vi "Swerve Drive.vi"(5 "Rot. Point X":dbl, 6 "Auto Controls":bool, 7 "Rot. Point Y":dbl) -> ()   [LabVIEW 2020]
uses:
  Robot Global Data.vi
  <vilib>/addons/control/pid/pid.llb/PID (DBL).vi
  <vilib>/addons/control/pid/NI_PID_pid.lvlib
panel:
  out "Gyro Angle":dbl(knob)=-0.120849609375 scale=0.0..360.0
  out "Heading":dbl=-0.60150146484375
  in  "Maintain Z Angle PID gains":T1={"proportional gain (Kc)"=0.0045, "integral time (Ti, min)"=0.0, "derivative time (Td, min)"=0.0} {"derivative time (Td, min)" format="%.4f"; "integral time (Ti, min)" format="%.4f"; "proportional gain (Kc)" format="%.4f"}
  in  "FeedForward":dbl
  in  "fr offset":dbl(knob)=326.0 scale=-180.0..180.0
  in  "fl offset":dbl(knob)=182.3 scale=-180.0..180.0
  in  "br offset":dbl(knob)=52.0 scale=-180.0..180.0
  in  "bl offset":dbl(knob)=358.0 scale=-180.0..180.0
  in  "Robot Length":dbl=25.0
  in  "Robot Width":dbl=25.0
  # "Comp bot\nFL: -2\nFR: -2\nBL: -1\nBR: 0"
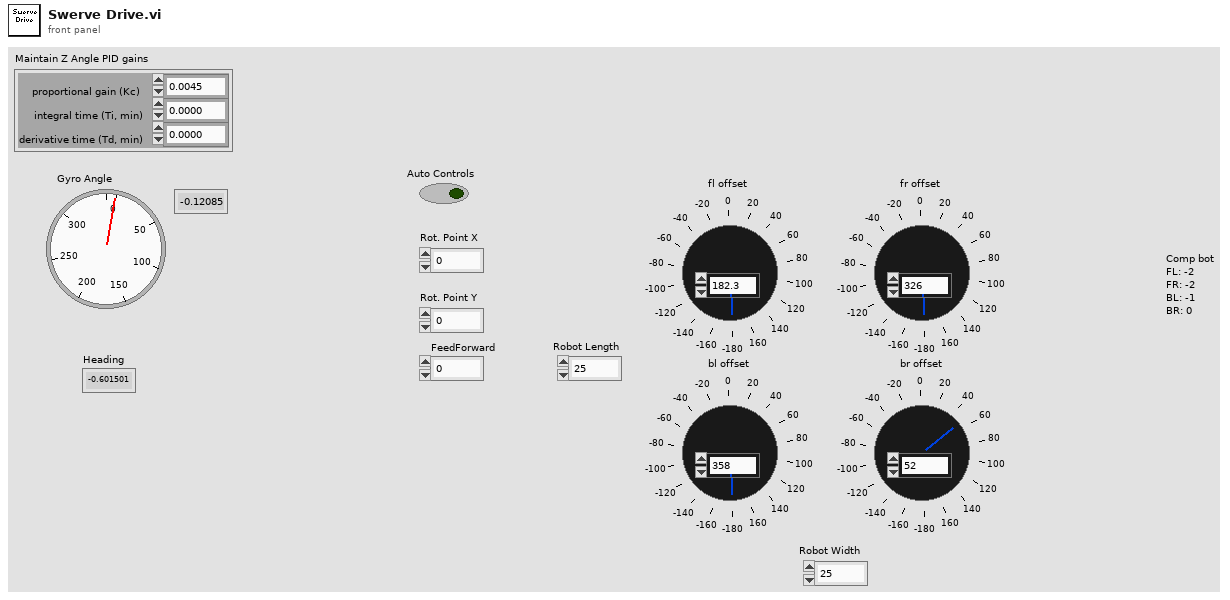
[diagram p1: front panel]
types:
  T1 = cluster{"proportional gain (Kc)":dbl, "integral time (Ti, min)":dbl, "derivative time (Td, min)":dbl}
  T2 = enum16{"Back Left", "Back Right", "Front Left", "Front Right"}
  T3 = typedef "WPI_MotorControlDeviceRef.ctl" = cluster{"DeviceStatus":errorcluster, "Type":T4, "PWM":cluster{"PWM Channel":T5, "DeadBand":T6}, "CAN":cluster{"Device Number":u8, "SetOutput VI Ref":variant, "GetOutput VI Ref":variant, "Enable VI Ref":variant, "Disable VI Ref":variant, "Data":variant}, "Invert":bool, "DIO PWM":cluster{"PWM \"Enable\" Channel":T5, "DIOChannel":T7, "PWM Rate":dbl}}
  T4 = typedef "WPI_MotorControlType.ctl" = enum16{"PWM", "CAN", "DIO PWM"}
  T5 = typedef "FPGA_DIOPWMChannel.ctl" = enum8{"PWM 0", "PWM 1", "PWM 2", "PWM 3", "PWM 4", "PWM 5", "PWM 6", "PWM 7", "PWM 8", "PWM 9", "PWM MXP 0", "PWM MXP 1", "PWM MXP 2", "PWM MXP 3", "PWM MXP 4", "PWM MXP 5", "PWM MXP 6", "PWM MXP 7", "PWM MXP 8", "PWM MXP 9", "Invalid"}
  T6 = typedef "WPI_PWMDeadband.ctl" = cluster{"Name":string, "maxPositivePwm":i32, "minPositivePwm":i32, "centerPwm":i32, "maxNegativePwm":i32, "minNegativePwm":i32, "angularRange":u16}
  T7 = typedef "FPGA_DIOChannel.ctl" = enum8{"DIO 0", "DIO 1", "DIO 2", "DIO 3", "DIO 4", "DIO 5", "DIO 6", "DIO 7", "DIO 8", "DIO 9", "DIO MXP 0", "DIO MXP 1", "DIO MXP 2", "DIO MXP 3", "DIO MXP 4", "DIO MXP 5", "DIO MXP 6", "DIO MXP 7", "DIO MXP 8", "DIO MXP 9", "DIO MXP 10", "DIO MXP 11", "DIO MXP 12", "DIO MXP 13", "DIO MXP 14", "DIO MXP 15", "SPI Port CS1", "SPI Port CS2", "SPI Port CS3", "SPI Port MISO", "SPI Port MOSI", "Invalid"}
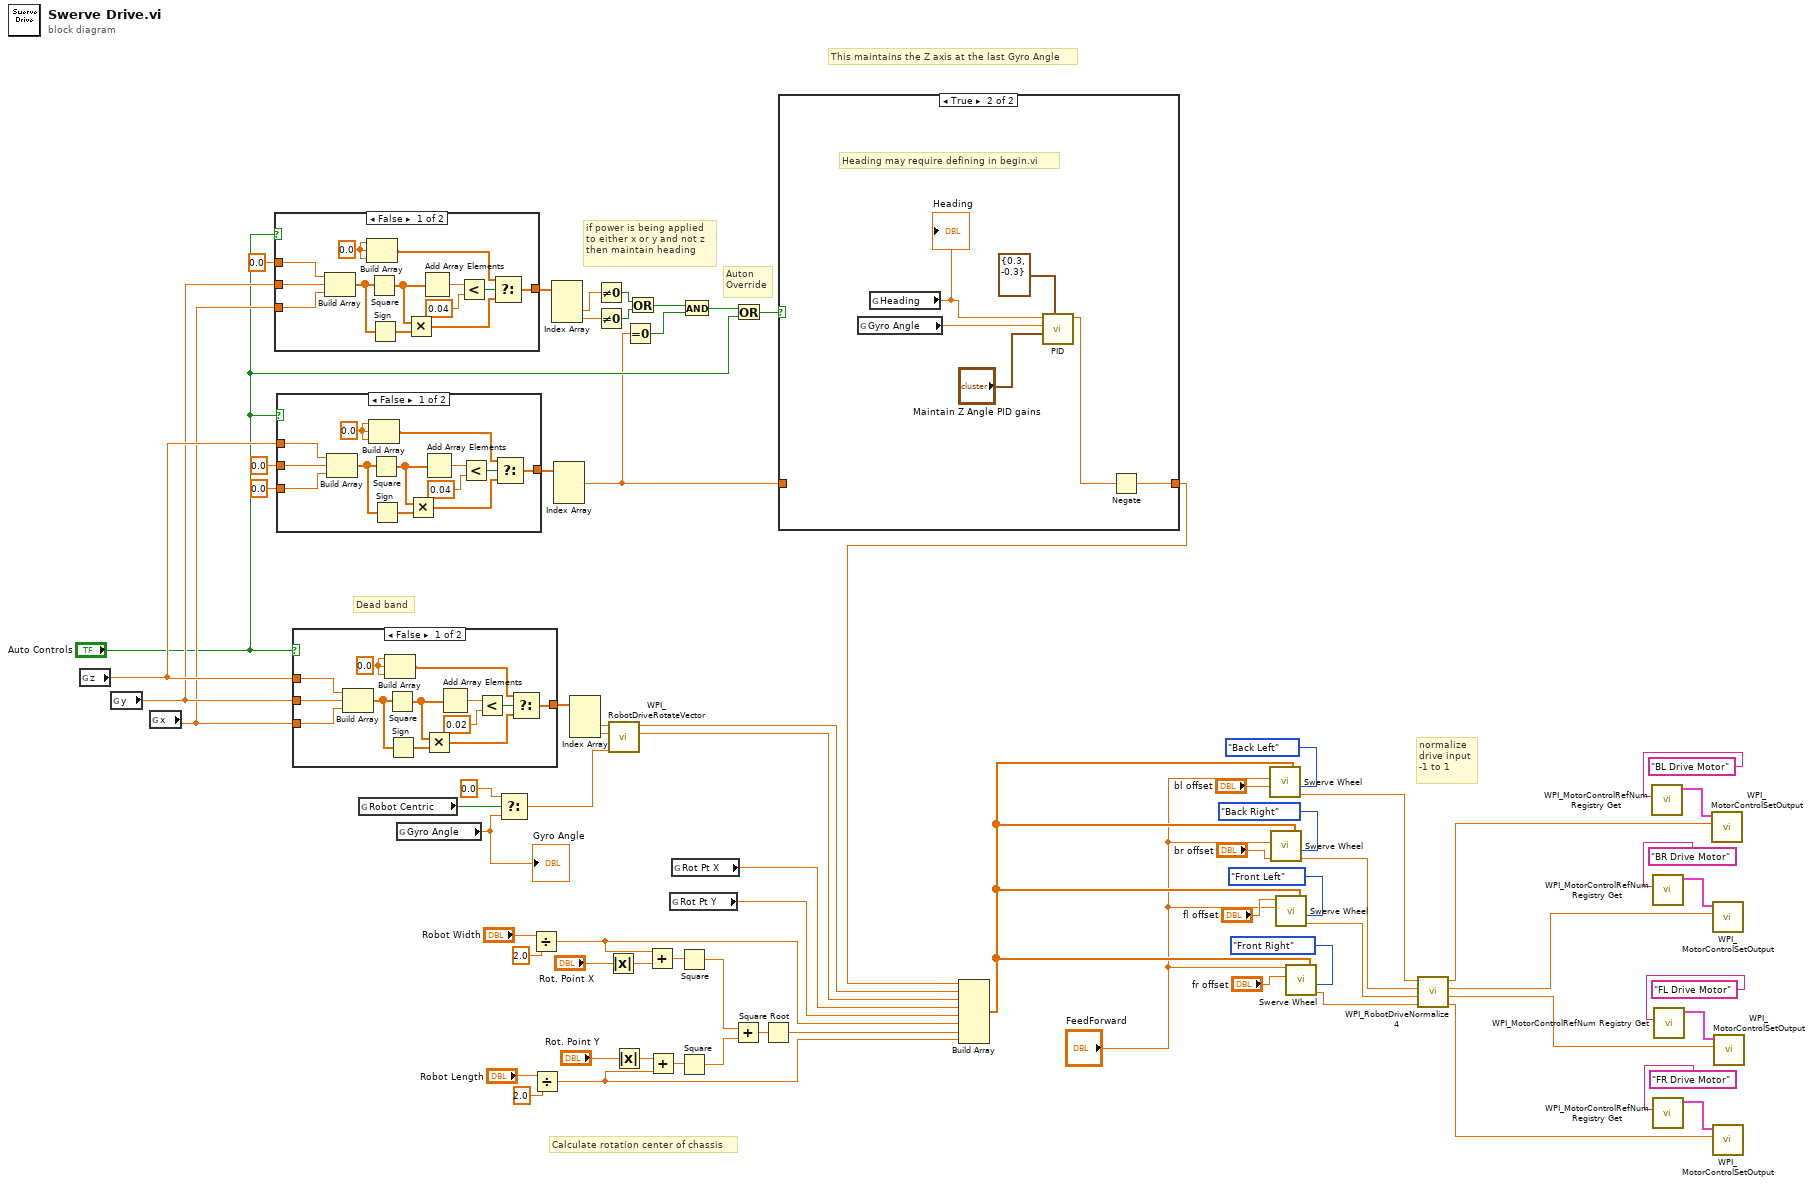
[diagram p0: block diagram]
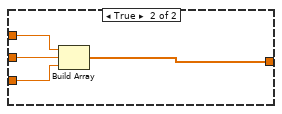
[diagram p2: hidden frame]
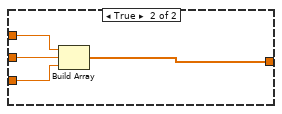
[diagram p3: hidden frame]
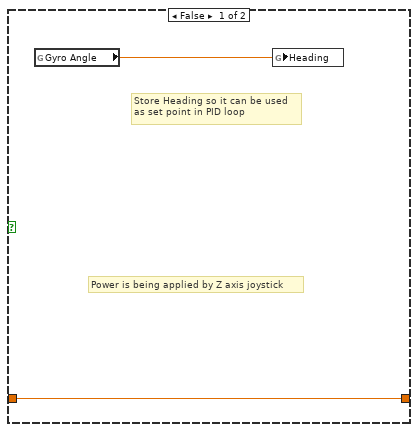
[diagram p4: hidden frame]
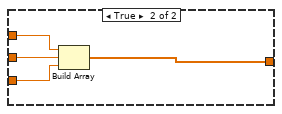
[diagram p5: hidden frame]
diagram:
  # "Auton\nOverride"
  # "This maintains the Z axis at the last Gyro Angle"
  # "if power is being applied\nto either x or y and not z\nthen maintain heading"
  # "normalize\ndrive input\n-1 to 1"
  # "Calculate rotation center of chassis"
  # "Dead band"
  n1 = global read "Robot Global Data.vi" "z"() -> (w24:dbl)
  n2 = global read "Robot Global Data.vi" "y"() -> (w20:dbl)
  n3 = global read "Robot Global Data.vi" "x"() -> (w19:dbl)
  n4 = case shown="False" "Auto Controls" {
    tunnel: w20 -> [w73 w88]
    tunnel: w19 -> [w77 w89]
    tunnel: 0.0 ("z") -> [w74 w86]
    tunnel: [w75 w87] -> w22
    frame False {
      w81 = 0.0 ("element")
      n5 = Build Array(w74, w73, w77) -> (w80:dbl[])
      n6 = Build Array(w81, w81, w81) -> (w82:dbl[])
      n7 = Square(x=w80) -> (x^2=w78:dbl[])
      n8 = Sign(1:w80) -> (0:w79:dbl[])
      n9 = Multiply(x=w78, y=w79) -> (x*y=w76:dbl[])
      n10 = Add Array Elements(numeric array=w78) -> (sum=w85:dbl)
      n11 = Less?(x=w85, y=0.04 ("x")) -> (x < y?=w83:bool)
      n12 = Select(t=w82, s=w83, f=w76) -> (s? t:f=w75:dbl[])
    }
    frame True {
      n13 = Build Array(w86, w88, w89) -> (w87:dbl[])
    }
  }
  n14 = case shown="False" "Auto Controls" {
    tunnel: 0.0 ("y") -> [w90 w105]
    tunnel: 0.0 ("x") -> [w94 w106]
    tunnel: w24 -> [w91 w103]
    tunnel: [w92 w104] -> w23
    frame False {
      w98 = 0.0 ("element")
      n15 = Build Array(w91, w90, w94) -> (w97:dbl[])
      n16 = Build Array(w98, w98, w98) -> (w99:dbl[])
      n17 = Square(x=w97) -> (x^2=w95:dbl[])
      n18 = Sign(1:w97) -> (0:w96:dbl[])
      n19 = Multiply(x=w95, y=w96) -> (x*y=w93:dbl[])
      n20 = Add Array Elements(numeric array=w95) -> (sum=w102:dbl)
      n21 = Less?(x=w102, y=0.04 ("x")) -> (x < y?=w100:bool)
      n22 = Select(t=w99, s=w100, f=w93) -> (s? t:f=w92:dbl[])
    }
    frame True {
      n23 = Build Array(w103, w105, w106) -> (w104:dbl[])
    }
  }
  n24 = case shown="False" "Auto Controls" {
    tunnel: w20 -> [w108 w122]
    tunnel: w19 -> [w112 w123]
    tunnel: w24 -> [w109 w120]
    tunnel: [w110 w121] -> w68
    frame False {
      w116 = 0.0 ("element")
      n25 = Build Array(w109, w108, w112) -> (w115:dbl[])
      n26 = Build Array(w116, w116, w116) -> (w117:dbl[])
      n27 = Square(x=w115) -> (x^2=w113:dbl[])
      n28 = Sign(1:w115) -> (0:w114:dbl[])
      n29 = Multiply(x=w113, y=w114) -> (x*y=w111:dbl[])
      n30 = Add Array Elements(numeric array=w113) -> (sum=w119:dbl)
      n31 = Less?(x=w119, y=0.02 ("x")) -> (x < y?=w107:bool)
      n32 = Select(t=w117, s=w107, f=w111) -> (s? t:f=w110:dbl[])
    }
    frame True {
      n33 = Build Array(w120, w122, w123) -> (w121:dbl[])
    }
  }
  n34 = global read "Robot Global Data.vi" "Robot Centric"() -> (w67:bool)
  n35 = global read "Robot Global Data.vi" "Gyro Angle"() -> (w65:dbl)
  "Gyro Angle" <- w65
  n36 = Select(t=0.0, s=w67, f=w65) -> (s? t:f=w62:dbl)
  n37 = Divide(x="Robot Width", y=2.0) -> (x/y=w47:dbl)
  n38 = Divide(x="Robot Length", y=2.0) -> (x/y=w49:dbl)
  n39 = Index Array(array=w22) -> (element #2=w18:dbl, element #3=w6:dbl)  [unwired: 3 in, 1 out]
  n40 = Index Array(array=w23) -> (element #1=w3:dbl)  [unwired: 3 in, 2 out]
  n41 = Index Array(array=w68) -> (element #2=w64:dbl, element #3=w63:dbl)  [unwired: 3 in, 1 out]
  n42 = Not Equal To 0?(x=w18) -> (x != 0?=w5:bool)
  n43 = Not Equal To 0?(x=w6) -> (x != 0?=w4:bool)
  n44 = Absolute Value(x="Rot. Point X") -> (abs(x)=w61:dbl)
  n45 = call "WPI_RobotDriveRotateVector.vi"("Angle"=w62, "X"=w63, "Y"=w64) -> ("X'"=w44:dbl, "Y'"=w43:dbl)  [unwired: 7 in]
  n46 = Absolute Value(x="Rot. Point Y") -> (abs(x)=w59:dbl)
  n47 = Equal To 0?(x=w3) -> (x = 0?=w1:bool)
  n48 = Or(x=w5, y=w4) -> (x .or. y?=w2:bool)
  n49 = Add(x=w47, y=w61) -> (x+y=w60:dbl)
  n50 = Add(x=w59, y=w49) -> (x+y=w58:dbl)
  n51 = global read "Robot Global Data.vi" "Rot Pt Y"() -> (w46:dbl)
  n52 = global read "Robot Global Data.vi" "Rot Pt X"() -> (w45:dbl)
  n53 = Square(x=w60) -> (x^2=w56:dbl)
  n54 = Square(x=w58) -> (x^2=w57:dbl)
  n55 = And(x=w2, y=w1) -> (x .and. y?=w17:bool)
  n56 = Add(x=w56, y=w57) -> (x+y=w55:dbl)
  n57 = Or(x=w17, y="Auto Controls") -> (x .or. y?=w16:bool)
  n58 = Square Root(x=w55) -> (sqrt(x)=w48:dbl)
  n59 = case shown="True" w16 {
    tunnel: w3 -> [w124 _]
    tunnel: [w124 w126] -> w27
    frame False {
      # "Store Heading so it can be used\nas set point in PID loop"
      # "Power is being applied by Z axis joystick"
      n60 = global read "Robot Global Data.vi" "Gyro Angle"() -> (w125:dbl)
      n61 = global write "Robot Global Data.vi" "Heading"(w125) -> ()
    }
    frame True {
      # "Heading may require defining in begin.vi"
      n62 = global read "Robot Global Data.vi" "Gyro Angle"() -> (w130:dbl)
      n63 = global read "Robot Global Data.vi" "Heading"() -> (w129:dbl)
      "Heading" <- w129
      n64 = call-poly <vilib>:"PID.vi"("output range"=cluster{"output high":dbl, "output low":dbl} {"output high"=0.3, "output low"=-0.3}, "PID gains"="Maintain Z Angle PID gains", "process variable"=w130, "setpoint"=w129) -> ("output"=w127:dbl)  [unwired: 6 in, 1 out]
      n65 = Negate(x=w127) -> (-x=w126:dbl)
    }
  }
  n66 = Build Array(w27, w43, w44, w45, w46, w47, w48, w49) -> (w32:dbl[])
  n67 = call "Swerve Wheel.vi"("Wheel"=T2."Back Left", "FeedForward"="FeedForward", "Inputs"=w32, "bl offset"="bl offset") -> ("Speed"=w40:dbl)  [unwired: 3 in]
  n68 = call "Swerve Wheel.vi"("Wheel"=T2."Back Right", "FeedForward"="FeedForward", "Inputs"=w32, "br offset"="br offset") -> ("Speed"=w35:dbl)  [unwired: 3 in]
  n69 = call "Swerve Wheel.vi"("Wheel"=T2."Front Left", "FeedForward"="FeedForward", "Inputs"=w32, "fl offset"="fl offset") -> ("Speed"=w34:dbl)  [unwired: 3 in]
  n70 = call "Swerve Wheel.vi"("Wheel"=T2."Front Right", "FeedForward"="FeedForward", "Inputs"=w32, "fr offset"="fr offset") -> ("Speed"=w33:dbl)  [unwired: 3 in]
  n71 = call "WPI_RobotDriveNormalize 4.vi"("D"=w33, "C"=w34, "B"=w35, "A"=w40) -> ("D'"=w69:dbl, "C'"=w70:dbl, "B'"=w71:dbl, "A'"=w72:dbl)
  n72 = call <vilib>:"WPI_MotorControlRefNum Registry Get.vi"("refnum name"="BL Drive Motor") -> ("MotorControlDevRef"=w15:T3)  [unwired: 9 in, 1 out]
  n73 = call <vilib>:"WPI_MotorControlRefNum Registry Get.vi"("refnum name"="BR Drive Motor") -> ("MotorControlDevRef"=w14:T3)  [unwired: 9 in, 1 out]
  n74 = call <vilib>:"WPI_MotorControlRefNum Registry Get.vi"("refnum name"="FR Drive Motor") -> ("MotorControlDevRef"=w12:T3)  [unwired: 9 in, 1 out]
  n75 = call <vilib>:"WPI_MotorControlRefNum Registry Get.vi"("refnum name"="FL Drive Motor") -> ("MotorControlDevRef"=w13:T3)  [unwired: 9 in, 1 out]
  n76 = call <vilib>:"WPI_MotorControlSetOutput.vi"("Output"=w72, "MotorControlDevRef"=w15) -> ()  [unwired: 7 in, 3 out]
  n77 = call <vilib>:"WPI_MotorControlSetOutput.vi"("Output"=w71, "MotorControlDevRef"=w14) -> ()  [unwired: 7 in, 3 out]
  n78 = call <vilib>:"WPI_MotorControlSetOutput.vi"("Output"=w69, "MotorControlDevRef"=w12) -> ()  [unwired: 7 in, 3 out]
  n79 = call <vilib>:"WPI_MotorControlSetOutput.vi"("Output"=w70, "MotorControlDevRef"=w13) -> ()  [unwired: 7 in, 3 out]
